vi "Pitch_LFO_SubVI.vi"(0 "Note Frequency":dbl, 2 "Ammount":dbl, 3 "Rate":dbl) -> (7 "Note Pitch":waveform(dbl))   [LabVIEW 2024]
uses:
  <vilib>/measure/NI_MABase.lvlib
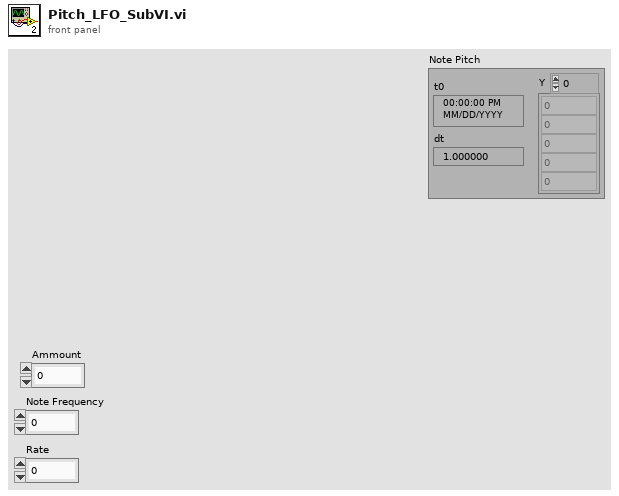
[diagram p1: front panel]
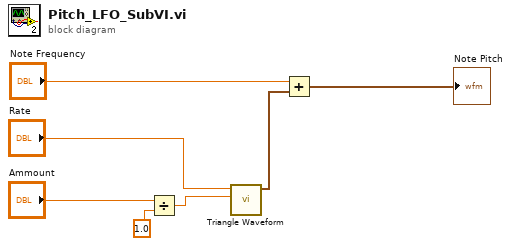
[diagram p0: block diagram]
diagram:
  n1 = Divide(x="Ammount", y=1.0) -> (x/y=w4:dbl)
  n2 = call <vilib>:"Triangle Waveform.vi"("amplitude"=w4, "frequency"="Rate") -> ("signal out"=w2:waveform(dbl))  [unwired: 8 in, 1 out]
  n3 = Add(x="Note Frequency", y=w2) -> (x+y=→"Note Pitch":waveform(dbl))
